vi "General Controller with DSA.vi"() -> ()   [LabVIEW 2013]
uses:
  <vilib>/Simulation/Scripting/Companion Diagram/SimConfigNode/SimParams.ctl
  <vilib>/Simulation/Scripting/Companion Diagram/SimConfigNode/_simSolvers.ctl
  <vilib>/Simulation/Implementation/Shared/SIMSCR Execution Mode.ctl
  <vilib>/Platform/TimedLoop/XDataNode/timing_clust.ctl
  <vilib>/Platform/TimedLoop/XDataNode/nitl_modes.ctl
  <vilib>/Platform/TimedLoop/XDataNode/wakeup.ctl
  <vilib>/Simulation/Param Hierarchy/Typedefs/SIMPH Param Control Actions.ctl
  <vilib>/Simulation/Implementation/Shared/SIM limit type.ctl
  <vilib>/Simulation/Implementation/Shared/NILVSim_ParamChanged.vi
  <vilib>/Simulation/Implementation/Shared/NILVSim_FinishedLate.vi
  <vilib>/Simulation/Implementation/Shared/NILVSIM_BeginStep.vi
  <vilib>/Simulation/Utility/Implementation/SIM Halt.vi
  <vilib>/Simulation/Utility/Implementation/SIM SimulationParams.vi
  <vilib>/Simulation/DataSources/Implementation/NILVSim Signal Generator.llb/SIM Signal Generator (scalar).vi
  <vilib>/Simulation/SignalArithmetic/Implementation/NILVSim Gain.llb/SIM Gain (scalar).vi
  <vilib>/Simulation/ContinuousLinear/Implementation/NILVSim Integrator new.llb/SIM Integrator distributor (scalar).vi
  <vilib>/Simulation/Implementation/Shared/SIM Is Init or Final Stage.vi
  <vilib>/Simulation/ContinuousLinear/Implementation/NILVSim Integrator new.llb/SIM Integrator collector (scalar).vi
  <vilib>/Simulation/ContinuousLinear/Implementation/NILVSim Transfer Function Direct.llb/SIM Transfer Function Direct (SISO).vi
  <vilib>/Simulation/SignalDisplay/Implementation/NILVSim Time Waveform.llb/SIM Time Waveform (vector).vi
  <vilib>/Simulation/Implementation/Shared/NILVSim_Manager.vi
  <vilib>/Simulation/Implementation/Shared/NILVSim_FinalizeModel.vi
  <vilib>/myRIO/Instrument Drivers/Onboard IO/AO/vis/Smart Open.vi
  <vilib>/myRIO/Instrument Drivers/Onboard IO/AO/vis/Write.vi
  <vilib>/myRIO/Instrument Drivers/Onboard IO/AI/vis/Smart Open.vi
  <vilib>/myRIO/Instrument Drivers/Onboard IO/AI/vis/Read.vi
  <vilib>/Simulation/Utility/Implementation/NILVSim SimulationParams (core).vi
  <vilib>/myRIO/Instrument Drivers/Onboard IO/AO/vis/Open.vi
  <vilib>/myRIO/Instrument Drivers/Onboard IO/AI/vis/Open.vi
  <vilib>/myRIO/Common/Instrument Driver Framework/myRIO v1.0/AO/vis/myRIO v1.1 Open AO.vi
  <vilib>/myRIO/Common/Instrument Driver Framework/myRIO v1.0/AI/vis/myRIO v1.1 Open AI.vi
  <vilib>/myRIO/Common/Instrument Driver Framework/Utilities/vis/Validate Channels.vi
  <vilib>/myRIO/Common/Instrument Driver Framework/myRIO v1.0/AO/vis/myRIO v1.0 Reserve AO.vi
  <vilib>/myRIO/Common/Instrument Driver Framework/myRIO v1.0/AI/vis/myRIO v1.0 Reserve AI.vi
  <vilib>/myRIO/Common/Instrument Driver Framework/myRIO v1.0/AO/vis/myRIO v1.0 Build MUX Configuration AO.vi
  <vilib>/myRIO/Common/Instrument Driver Framework/myRIO v1.0/Resource Manager/vis/myRIO v1.0 Reserve Channel List.vi
  <vilib>/myRIO/Common/Instrument Driver Framework/myRIO v1.0/AI/vis/myRIO v1.0 Build MUX Configuration AI.vi
  <vilib>/myRIO/Common/Instrument Driver Framework/myRIO v1.0/Resource Manager/vis/myRIO v1.0 Reserve Channel.vi
  <vilib>/myRIO/Common/Instrument Driver Framework/myRIO v1.0/Resource Manager/vis/myRIO v1.0 Unreserve Channel.vi
  <vilib>/myRIO/Common/Instrument Driver Framework/myRIO v1.0/Resource Manager/vis/myRIO v1.0 Build Mutex Name.vi
  <vilib>/myRIO/Common/Instrument Driver Framework/myRIO v1.0/myRIO v1.1 Open.vi
  <vilib>/myRIO/Common/Instrument Driver Framework/myRIO v1.0/AO/vis/myRIO v1.0 Get Scaling Constants AO.vi
  <vilib>/Utility/VariantDataType/GetNumericInfo.vi
  <vilib>/Utility/error.llb/Error Cluster From Error Code.vi
  <vilib>/myRIO/Common/Instrument Driver Framework/Utilities/vis/IO Manager.vi
  <vilib>/myRIO/Common/Instrument Driver Framework/Utilities/vis/Configuration Manager.vi
  <vilib>/myRIO/Common/Instrument Driver Framework/myRIO v1.0/myRIO v1.0 Close.vi
  <vilib>/myRIO/Common/Instrument Driver Framework/myRIO v1.0/AO/vis/myRIO v1.0 Write AO.vi
  <vilib>/Simulation/Implementation/Shared/SIM Unbundle Sim Info.vi
  <vilib>/Utility/error.llb/Clear Errors.vi
  <vilib>/Simulation/Implementation/Shared/NILVSim_GetModelError.vi
  <vilib>/Simulation/Implementation/Shared/SIM Bundle Sim Info.vi
  <vilib>/Simulation/Implementation/Shared/SIMSH Read Queue.vi
  <vilib>/Simulation/Implementation/Shared/NILVSim_Initialize.vi
  <vilib>/Simulation/Utility/Implementation/NILVSim Get Time and IsAcceptedStep.vi
  SubVIs/Dropable_DSA.vi
  <vilib>/myRIO/Common/Instrument Driver Framework/myRIO v1.0/AI/vis/myRIO v1.0 Get Scaling Constants AI.vi
  <vilib>/myRIO/Common/Instrument Driver Framework/myRIO v1.0/AI/vis/myRIO v1.0 Read AI.vi
  <vilib>/Simulation/Scripting/Companion Diagram/SimConfigNode/SimDog.xnode
  <vilib>/Platform/TimedLoop/XDataNode/XDataNode.xnode
  <vilib>/Simulation/Implementation/XNodeFramework/SimXNode/SimX.xnode
  <vilib>/Simulation/ContinuousLinear/Implementation/NILVSim Integrator new.llb/SIM Integrator (scalar).vi
  <vilib>/Platform/TimedLoop/XDataNode/XDNodeRunTimeDep.lvlib
  <vilib>/Simulation/Implementation/Shared/NI_SIM_Implementation.lvlib
panel:
  in  "Tab Control":T1(tab)=enum."DSA"
  out "Scope":waveform(dbl)[](graph)=[{"t0"=timestamp(335.31 s since 1904-01-01), "dt"=1.0, "Y"=[0.0]}, {"t0"=timestamp(335.31 s since 1904-01-01), "dt"=1.0, "Y"=[-3.1279355385042793]}, {"t0"=timestamp(335.31 s since 1904-01-01), "dt"=1.0, "Y"=[10.0]}]
  in  "ON? 2":bool
  in  "alpha":dbl=10.0
  in  "Td":dbl=0.003
  in  "Offset 2":dbl
  in  "ON?":bool
  in  "Kp":dbl=1.0
  in  "Lower":dbl=-5.0
  in  "Upper":dbl=5.0
  in  "Ti":dbl=0.16
  in  "Signal Type":u16(ring)=1 items=["Sine", "Square", "Sawtooth", "Random"]
  in  "Offset":dbl
  in  "Amplitude":dbl
  in  "Frequency":dbl=0.5
  out "Bode Magnitude":cluster{dbl[], dbl[]}(graph)={[1.0, 1.2689610031679222, 1.6102620275609394, 2.043359717856942, 2.592943797404667, 3.2903445623126686, 4.1753189365604015, 5.298316906283708, 6.7233575364993365, 8.531678524172808, 10.826367338740546, 13.73823795883263, 17.43328822199988, 22.122162910704493, 28.072162039411772, 35.62247890262442, 45.20353656360243, 57.36152510448679, 72.7895384398315, 92.36708571873861, 117.21022975334806, 148.73521072935117, 188.73918221350976, 239.5026619987486, 303.9195382313198, 385.6620421163472, 489.3900918477494, 621.0169418915616, 788.0462815669912, 1000.0], [1.0018651131002922, 1.0016050465725763, 1.0010062349698785, 1.0002931137870483, 0.9991459144089636, 0.9972202532472595, 0.9944020144562293, 0.9903082002861369, 0.983855401702225, 0.9738705481650444, 0.9582906977613652, 0.9358034848813956, 0.9036393454169751, 0.857649976648417, 0.7964400088413218, 0.7217565791716765, 0.6359239660806931, 0.5476382842843324, 0.461415834347026, 0.38116988425483045, 0.3091314427820101, 0.2514928062528439, 0.20170891904461263, 0.15879614847289658, 0.127858110424497, 0.10171304349328705, 0.08081117825531599, 0.06376794604720305, 0.050469140870365095, 0.039745706120179934]}
  out "Bode Phase":cluster{dbl[], dbl[]}(graph)={[1.0, 1.2689610031679222, 1.6102620275609394, 2.043359717856942, 2.592943797404667, 3.2903445623126686, 4.1753189365604015, 5.298316906283708, 6.7233575364993365, 8.531678524172808, 10.826367338740546, 13.73823795883263, 17.43328822199988, 22.122162910704493, 28.072162039411772, 35.62247890262442, 45.20353656360243, 57.36152510448679, 72.7895384398315, 92.36708571873861, 117.21022975334806, 148.73521072935117, 188.73918221350976, 239.5026619987486, 303.9195382313198, 385.6620421163472, 489.3900918477494, 621.0169418915616, 788.0462815669912, 1000.0], [-1.4001864556390353, -1.7425257743205063, -2.2774811113746067, -2.940300047591337, -3.797024621582645, -4.874740361894845, -6.244214499985965, -7.9488896703659435, -10.107416371370137, -12.8129960492024, -16.195047872218314, -20.2121008365249, -24.982209581081694, -30.62002310970157, -36.70295501035055, -43.18506539585506, -49.773026506300724, -56.0120451118291, -61.68921924132383, -66.61507141784128, -71.21117465500357, -75.07757805867544, -77.49128997241446, -81.82799122918105, -82.40583459630555, -84.09391534817092, -87.5421411007668, -88.23137376055858, -91.93060722680163, -98.46625820370649]}
  in  "Frequency Response":i32(slide)=1
  in  "START":bool
  in  "Excitation Specs":T2={"Initial Frequency"=1.0, "Final Frequency"=100.0, "Number of Frequencies"=30, "DSA Samping Time [s]"=0.001, "Amplitude [V]"=1.0, "Offset [V]"=0.0, "Freq Unit"=TRUE}
  in  "Cycle Specs":T3={"Cycles To Settle (M)"=5, "Cycles To Calculate (N)"=5}
  out "Running":bool
  out "FINISHED LATE":bool
  out "Stopped":bool=TRUE
  in  "STOP":bool
  out "Live Signals":cluster{"DSA Excitation":dbl, "output y(t)":dbl}(graph)={"DSA Excitation"=0.9745443172783077, "output y(t)"=-0.9745443172783077}
  in  "Exist Porgram":bool
  # "PMCL Generic Controller with DSA"
  # "Generic Controller"
  # "Controllers Implemenetation"
  # "Controllers"
  # "Reference  Signal"
  # "The Lead-Lag Controller has the form:"
  # "Proportional:"
  # "Intergrator Limits"
  # "Lag:"
  # "Note: Ti is the integrator time constant. Ti = 1/Ki"
  # "Lead:"
  # "Note: When using the DSA, set this amplitude to 0!"
  # "Note: Td is the lag compensator time constant."
  # "Dynamic Signal Analyzer"
  # "Magnitude"
  # "Controls"
  # "Operation"
  # "Frequency Response"
  # "Plant"
  # "Return Ratio"
  # "Closed Loop"
  # "Phase"
  # "__"
  # "__"
  # "__"
  # "Excitation Frequencies"
  # "Frequency\nUnits"
  # "[Hz]"
  # "Excitation Magnitude"
  # "[rad/s]"
  # "Running the Program\n \n(1) Set the DSA Sampling Time, the rate at which the myRIO collects data and updates the control \n      effort sent to the plant.\n\n      - Note:   Sampling Rate = 1/(DSA Sampling Time)     where the default is 0.005 sec which \n                                                                                                              is a sampling rate of 200 Hz.\n \n      - Note: If the FINISHED LATE button flashes, the myRIO needs to sample at a slower rate.\n \n      - If you update the Controller Sampling Time, exist and rerun the program! Unlike the \n         Stand-Alone DSA program, the program's time step cannot be updated while it is running.\n \n \n(2) Press the white arrow above,          , to start the program.\n \n(3) Use the program. See Running the Controller, Running the DSA, and or Collecting Data.\n \n(4)  Click EXIT PROGRAM in the upper right hand corner to stop the progam."
  # "Running the DSA\n \n(1) Make sure the closed loop system is STABLE with the given controller being used!\n \n(2) Turn off the reference signal (set the amplitude = 0).\n \n(3) Select the response to be measured: Plant, Return Ratio, or Closed Loop Response.\n\n(4) Set other desired parameters: \n\n      - Inital Frequency: Atleast 1 decade before frequency of interest\n\n      - Final Frequency: Atleast 1 decade before frequency of interest\n \n             ~ Note:  Max Final Frequency = Sampling Rate/2  where for this case would be 1.25 kHz.          \n\n      - Number of Frequnecies: 30\n\n      - Amplitude: Largest Amplitude such that the control effort does not staturate\n\n      - Cycles to Settle: 5 minimum for low frequencies & 20 minimum for high frequencies\n\n      - Cycles to Calculate: 5 minimum for low frequencies & 20 minimum for high frequencies  \n\n(5) Press START to start the DSA.\n\n(6) Press STOP to stop the DSA if needed or it will stop when it is finished."
  # "Running the Controller\n \n(1) Adjust the Lead-Lag Compensator controller's inputs to their desired values.\n\n(2) Adjust the reference signal's inputs to their desired values.\n \n      - NOTE: To turn off the refence signal, set the amplitude of the refence signal to zero!"
  # "Collecting Data\n \n(1) Right click the graph and select Export.\n \n      - NOTE: You can only record what is shown on the graph!\n\n(2) Choose the format you want to export your data to.\n \n       - Export Data To Clipboard: Copies it so you can paste it into a program like Matlab\n \n       - Export Data To Excel: Opens up your data in Excel.\n \n       - Export Simpliefed Image... : Saves your data as a cleaned up screenshot picture\n  \n Changing What You Record\n \nTo change the length of time displayed on the graph and thus the length of time you record data for, right click and select Chart History Length while the porgram is NOT running. \n \n        Chart History Length = (Desired Length of Time in Sec) / (Controller Sampling Time)"
  # "Wiring Details\n  \n       - AO 0:   System Reference\n \n       - AI   0+: Control Effort (Plant Input)\n       - AI   0- : AGND\n \n       - AI   1+: Plant / Sensor Output \n       - AI   1- : AGND\n\n   Notes:\n \n      - Ideally you would want AI 1+ to be the plant output. However as the plant output is not \n         always  a voltage, this will often be a sensor output. As a result, the measured frequency \n         response (bode plots) would be gained by the gain of the sensor.\n \n              ~ Usually the gain of the sensor is a constant though so just divide the magnitude values  \n                  by it."
  # "A DSA, or Dynamic Signal Analyzer is a tool that measures a the frequency response of a transfer function and plots its corresponding bode plots."
  # "A DSA works in 3 steps:\n\n      (1) It inputs a swept sine wave (a sine wave that increaes in frequency), D, at the feedback summing junction. This sine wave will show up through out the system with varying magnitudes and phase. It is how \n            the magnidute and phase of this swept sine wave changes is what we care about.\n\n      (2) It measures the signal at two points through out the system.\n\n      (3) It finds the frequency response of the  transfer function between the two points measured. This is easily shown as a bode plot as  the  magnidute of the frequency response is the magnitude of the signal \n           measured at one point divided the  magnitude of the singal at the other point and the phase of the frequency response is the phase of the signal measured at the first point minus the phase of the signal \n           measured at the second point.\n\n\nThe easiest way to explain this is to show how the DSA calculates the frequnecy response for a transfer function is to look how it does it for the 3 transfer functions we care about (plant, return ratio, and closed loop).\n\n      - Plant: The plant TF is just the ratio of the output of the plant to its input. Thus the DSA finds the frequency response of the plant TF by measuring the signal output by the plant (a swept sine wave), Y, and the \n                    signal input to the plant (a swept sine wave), C. Then it divides the magnitude of Y by the magnitude of C and subtracts the phase of C from the phase of Y at each frequency of the swept sine wave. This \n                     provides the frequency reponse of the plant as it changes with freqency.\n\n      - Return Ratio: The return ratio TF is just the ratio of the output of the loop to its input. Thus the DSA finds the frequency response of the return ratio TF by measuring the signal output by the loop (a swept sine \n                                 wave), M, and the signal input to the loop (a swept sine wave), E. Then it divides the magnitude of M by the magnitude of E and subtracts the phase of E from the phase of M at each frequency of \n                                 the swept sine wave. This provides the frequency reponse of the plant as it changes with freqency.\n\n      - Closed Loop: The closed loop TF is just the ratio of the output of the closed loop to its input. Thus the DSA finds the frequency response of the closed loop TF by measuring the signal output by the closed loop \n                                 (a swept sine  wave), Y, and the signal input to the closed loop (a swept sine wave), R. Then it divides the magnitude of Y by the magnitude of R and subtracts the phase of R from the phase of Y at \n                                  each frequency of the swept sine wave. This provides the frequency reponse of the plant as it changes with freqency."
  # "Copyright (c) 2015 Tyler Hamer\n\nPermission is hereby granted, free of charge, to any person obtaining a copy of this software and associated documentation files (the \"Software\"), to deal in the Software without restriction, including without limitation the rights to use, copy, modify, merge, publish, and/or distribute, but not sublicense, and/or sell copies of the Software, and to permit persons to whom the Software is furnished to do so, subject to the following conditions:\n\nThe above copyright notice and this permission notice shall be included in all copies or substantial portions of the Software.\n\nTHE SOFTWARE IS PROVIDED \"AS IS\", WITHOUT WARRANTY OF ANY KIND, EXPRESS OR IMPLIED, INCLUDING BUT NOT LIMITED TO THE WARRANTIES OF MERCHANTABILITY, FITNESS FOR A PARTICULAR PURPOSE AND NONINFRINGEMENT. IN NO EVENT SHALL THE AUTHORS OR COPYRIGHT HOLDERS BE LIABLE FOR ANY CLAIM, DAMAGES OR OTHER LIABILITY, WHETHER IN AN ACTION OF CONTRACT, TORT OR OTHERWISE, ARISING FROM, OUT OF OR IN CONNECTION WITH THE SOFTWARE OR THE USE OR OTHER DEALINGS IN THE SOFTWARE"
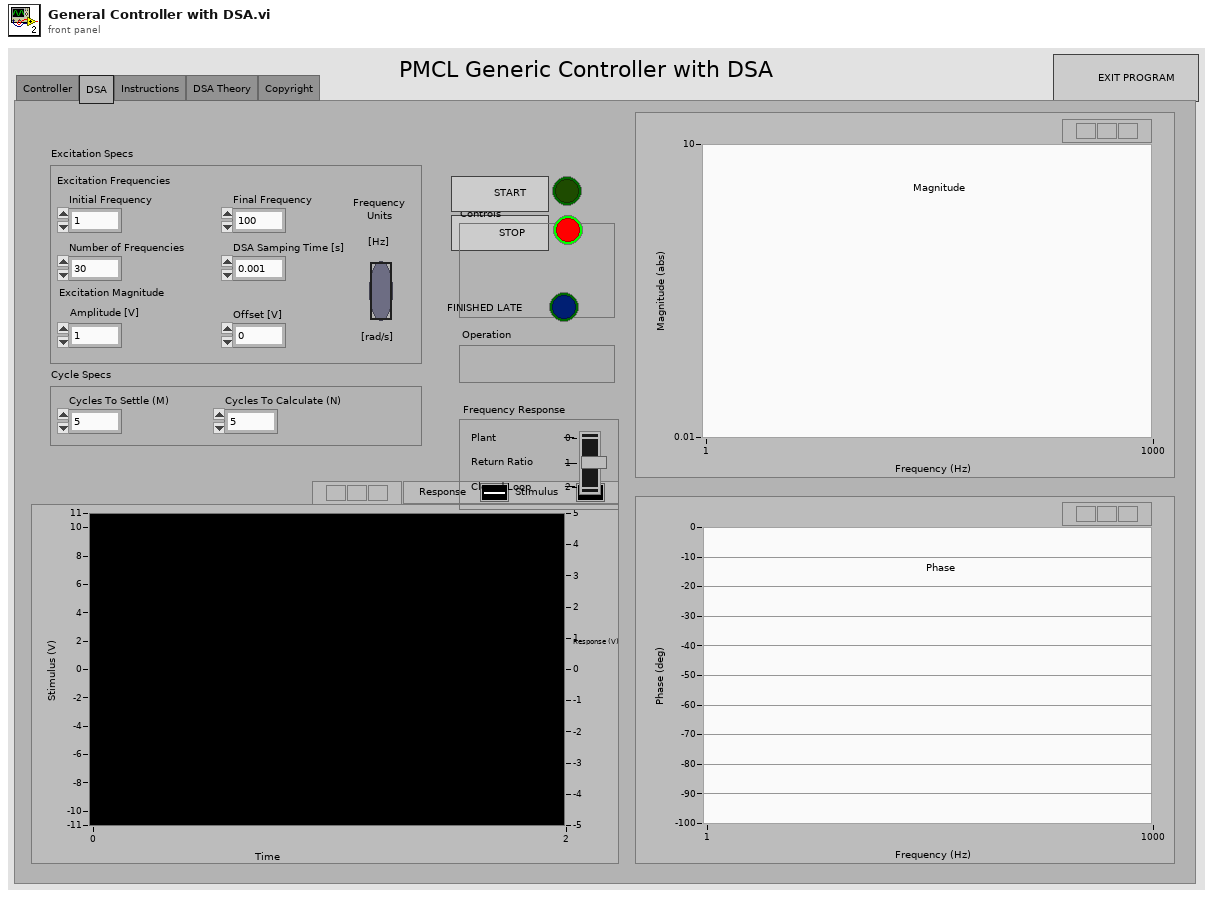
[diagram p1: front panel]
types:
  T1 = enum32{"Controller", "DSA", "Instructions", "DSA Theory", "Copyright"}
  T2 = cluster{"Initial Frequency":dbl, "Final Frequency":dbl, "Number of Frequencies":i16, "DSA Samping Time [s]":dbl, "Amplitude [V]":dbl, "Offset [V]":dbl, "Freq Unit":bool}
  T3 = cluster{"Cycles To Settle (M)":i16, "Cycles To Calculate (N)":i16}
  T4 = typedef "SIMSCR Execution Mode.ctl" = enum16{"Simulate to Completion", "Single Time-Step Simulation (Fixed Step Only)"}
  T5 = typedef "XDNodeRunTimeDep.lvlib/timing_clust.ctl" = cluster{"Expected End [f-1]":u64, "Actual End [f-1]":u64, "Finished Late? [f-1]":bool, "Expected End [i-1]":u64, "Actual End [i-1]":u64, "Finished Late? [i-1]":bool, "Expected Start [i]":u64, "Actual Start [i]":u64, "Expected Start [f]":u64, "Actual Start [f]":u64, "Source Name":string, "Structure Name":string, "Period":i64, "Deadline":i64, "Offset":i64, "Start":i64, "Priority":i32, "Timeout":i32, "Mode":T6, "Wakeup Reason":T7, "Error":errorcluster, "Source Type":string, "Secondary Source Type":string, "Global End Time":u64, "Global Start Time":u64, "Frame Duration":u64, "Iteration Duration":u64, "Assigned CPU":i32, "I/O Scan Engine Mode":u32}
  T6 = typedef "XDNodeRunTimeDep.lvlib/nitl_modes.ctl" = enum32{"No Change", "Process missed periods, maintain original phase", "Discard missed periods, maintain original phase", "Process missed periods, ignore original phase", "Discard missed periods, ignore original phase"}
  T7 = typedef "XDNodeRunTimeDep.lvlib/wakeup.ctl" = enum32{"Normal", "Aborted", "Asynchronous wakeup", "Timing source error", "Timed loop error", "Timeout"}
  T8 = typedef "SIMPH Param Control Actions.ctl" = enum16{"get params", "set params"}
  T9 = typedef "SIM limit type.ctl" = enum16{"upper", "lower", "both", "none"}
  T10 = typedef "SimParams.ctl" = cluster{"Initial Time (s)":dbl, "Final Time (s)":dbl, "Step Size (s)":dbl, "ODE Solver":T11, "Minimum Step Size (s)":dbl, "Maximum Step Size (s)":dbl, "Relative Tolerance":dbl, "Absolute Tolerance":dbl, "Software Timing":bool, "Initial Step Size (s)":dbl, "Automatic Fixed Step Size?":bool, "Automatic Discrete Step Size?":bool, "Discrete Step Size (s)":dbl, "Calculate using Time Step":bool, "Solver Wired?":bool, "Prev.Frm.Expected End":u64, "Prev.Frm.Actual End":u64, "Prev.Frm.Finished Late?":bool, "Prev.Iter.Expected End":u64, "Prev.Iter.Actual End":u64, "Prev.Iter.Finished Late?":bool, "Expected Iteration Start":u64, "Actual Iteration Start":u64, "Expected Frame Start":u64, "Actual Frame Start":u64, "Source Name":string, "Name":string, "Period":i64, "Deadline":i64, "Offset":i64, "Start":i64, "Priority":i32, "Timeout":i32, "Processor":i32, "Mode":enum32{"No Change", "Process missed periods, maintain original phase", "Discard missed periods, maintain original phase", "Process missed periods, ignore original phase", "Discard missed periods, ignore original phase"}, "Wakeup reason":enum32{"Normal", "Aborted", "Asynchronous wakeup", "Timing source error", "Timed loop error", "Timeout"}, "Error":errorcluster, "Source Type":string, "Secondary Source Type":string, "Global End Time":u64, "Global Start Time":u64, "Full Solver Reset":bool, "Execution Mode":T4, "Nan/Inf Check":bool, "Custom Solver Library":string, "Solver Is Variable":bool, "custom solver name":string, "Signal Collection Decimation":u32}
  T11 = typedef "_simSolvers.ctl" = enum16{"Runge-Kutta 1 (Euler)", "Runge-Kutta 2", "Runge-Kutta 3", "Runge-Kutta 4", "Runge-Kutta 23 (variable)", "Runge-Kutta 45 (variable)", "BDF (variable)", "Adams-Moulton (variable)", "Rosenbrock (variable)", "Discrete States Only", "SDIRK 4 (variable)", "Radau 5 (variable)", "Radau 9 (variable)", "Radau 13 (variable)", "Radau [Variable Order] (variable)", "Gear's Method (variable)", "Linearizer", "State Query", "Trim Eval", "Custom Solver"}
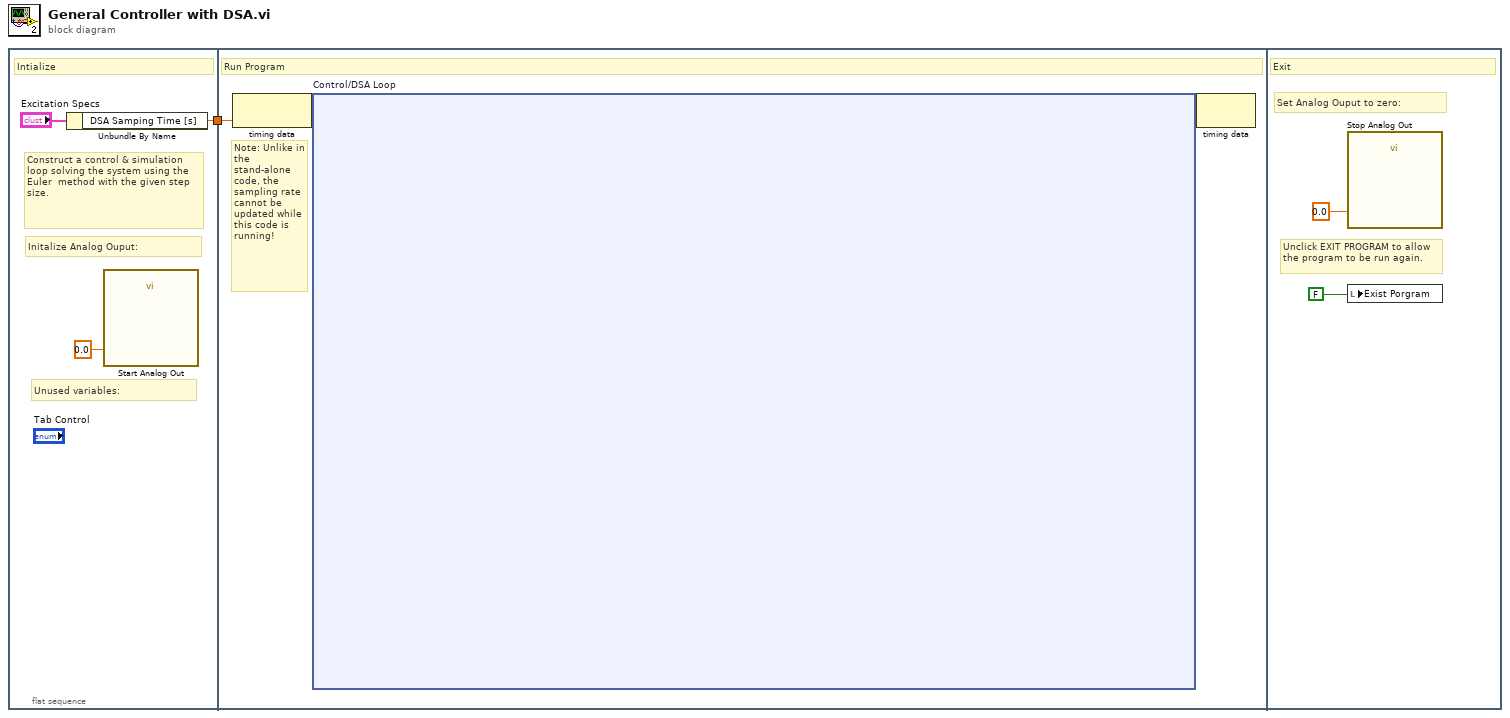
[diagram p0: block diagram]
diagram:
  n1 = flat-sequence {
    tunnel: [w2] -> w1
    tunnel: w1 -> [w5]
    frame #0 {
      # "Construct a control & simulation loop solving the system using the Euler  method with the given step size."
      # "Initalize Analog Ouput:"
      # "Unused variables:"
      # "Intialize"
      n2 = Unbundle By Name("Excitation Specs") -> ("DSA Samping Time [s]"=w2:dbl)
      n3 = call "Start Analog Out"("Vi (Control Effort) (C/AO0)"=0.0) -> ()  [unwired: 26 in, 1 out]
    }
    frame #1 {
      # "Note: Unlike in the stand-alone code, the sampling rate cannot be updated while this code is running!"
      # "Run Program"
      n4 = node-c288(w5) -> (w7:variant)
      n5 = node-c254 "Control/DSA Loop"(w7) -> (w6:variant)
      n6 = node-c288(w6) -> ()  [unwired: 1 out]
    }
    frame #2 {
      # "Unclick EXIT PROGRAM to allow the program to be run again."
      # "Set Analog Ouput to zero:"
      # "Exit"
      n7 = call "Stop Analog Out"("Vi (Control Effort) (C/AO0)"=0.0) -> ()  [unwired: 26 in, 1 out]
      n8 = local write "Exist Porgram"(FALSE) -> ()
    }
  }
